vi "Main.vi"(8 "error in (no error)":errorcluster, 11 "ModuleAdmin":refnum<class "ModuleAdmin.lvclass">) -> ()   [LabVIEW 2014, in "AppModule.lvlib"]
uses:
  AppModule.lvlib
  <userlib>/NIST/ModuleAdminLib/ModuleAdmin/ModuleAdmin.lvclass
  PublicAPI/Arguments/Requests/clStopArgument.ctl
  <userlib>/NIST/BaseClasses/BasePlugin_class/BasePlugin.lvclass/BasePlugin.ctl
  AppPlugins/AppPluginBaseClass/AppPluginsBase.lvclass
  <userlib>/NIST/ModuleAdminLib/ModuleAdmin/ModuleAdmin.lvclass/ModuleAdmin.ctl
  Framework/FrontPanel/TypeDefs/clEventConfig.ctl
  Modules/EventPlugins/EventPluginBaseClass/TypeDefs/clEvtReportArray.ctl
  Modules/EventPlugins/EventPluginBaseClass/TypeDefs/clEvtReport.ctl
  AppPlugins/AppPluginBaseClass/AppPluginsBase.lvclass/AppPluginsBase.ctl
  PublicAPI/Arguments/Requests/BC_AppInfo.ctl
  Framework/BusController/Admin/Registry/BCReg.lvclass
  <vilib>/Utility/error.llb/DialogType.ctl
  <userlib>/NIST/BaseClasses/BasePlugin_class/Accessors/Read PluginIniFilePath.vi
  <userlib>/NIST/BaseClasses/BasePlugin_class/Accessors/Write PluginIniFilePath.vi
  <userlib>/NIST/ModuleAdminLib/ModuleAdmin/Accessors/Write ShowPanel_.vi
  AppPlugins/AppPluginBaseClass/Accessors/Write clEvtReportArray.vi
  AppPlugins/AppPluginBaseClass/Accessors/Read clEvtReportArray.vi
  AppPlugins/AppPluginBaseClass/Accessors/Write BC_AppInfo.vi
  AppPlugins/AppPluginBaseClass/Accessors/Read BC_AppInfo.vi
  <userlib>/NIST/ModuleAdminLib/ModuleAdmin/Accessors/Read ShowPanel_.vi
  <userlib>/NIST/ModuleAdminLib/ModuleAdmin/Accessors/Read CloneRegRef.vi
  <vilib>/Utility/error.llb/Error Cluster From Error Code.vi
  <vilib>/ErrorRing/Error Ring.xnode
  <userlib>/NIST/ModuleAdminLib/CloneRegistration/CloneRegistration.lvclass
  <userlib>/NIST/ModuleAdminLib/ModuleAdmin.lvlib
  <userlib>/NIST/BaseClasses/Object_class/BaseObject.lvclass
  Modules/EventPlugins/EventPluginBaseClass/EventPluginBaseClass.lvclass
  Framework/Framework.lvlib
panel:
  out "error out":errorcluster
  # "This is the template for your cloneable module.\nYou should modifiy this to perform the functionality\nthat you want it to perform"
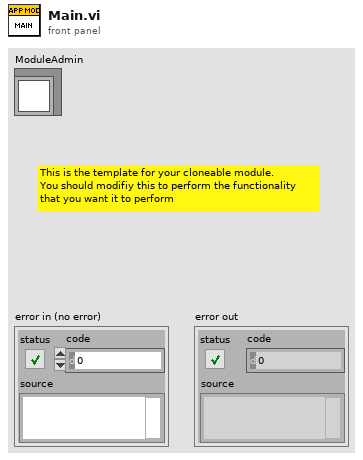
[diagram p1: front panel]
types:
  T1 = typedef "AppModule.lvlib/clRequestEvents.ctl" = cluster{"StopRequest":refnum<user-event>, "PathToINI":refnum<user-event>, " LoadPlugin":refnum<user-event>, "OpenAppConfig":refnum<user-event>, "WriteInputData":refnum<user-event>, "ReadInputData":refnum<user-event>, "GetAppOutput":refnum<user-event>, "WriteEvtConfig":refnum<user-event>, "WriteBcAppInfo":refnum<user-event>, "ReadBcAppInfo":refnum<user-event>, "AggregateRequest":refnum<user-event>, "WriteAppConfig":refnum<user-event>, "ReadAppConfig":refnum<user-event>, "CalcAppOutput":refnum<user-event>, "ShowPanel":refnum<user-event>}
  T2 = typedef "AppModule.lvlib/clBroadcastEvents.ctl" = cluster{"DidInit":refnum<user-event>, "StatusUpdate":refnum<user-event>, "ErrorReport":refnum<user-event>, "DidStop":refnum<user-event>, "PathToINI":refnum<user-event>, "InputData":refnum<user-event>, "OutputData":refnum<user-event>, "BcAppInfo":refnum<user-event>, "ConfigData":refnum<user-event>}
  T3 = typedef "AppModule.lvlib/clStopArgument.ctl" = cluster{"Exit via Stop Module Req?":bool, "Wait for Module to stop?":bool, "ModuleAdmin":refnum<class "ModuleAdmin.lvclass">}
  T4 = enum32{"Invalid", "Standard", "Closed", "Hidden", "Minimized", "Maximized"}
  T5 = typedef "Framework.lvlib/clEventConfig.ctl" = cluster{"UTC Time 0":timestamp, "Nominal Frequency":u16, "Reporting Rate":u16, "Fsamp":u32, "PosSeq":bool}
  T6 = typedef "EventPlugins.lvlib/EventPluginBaseClass.lvclass/clEvtReportArray.ctl" = T7[]
  T7 = typedef "EventPlugins.lvlib/EventPluginBaseClass.lvclass/clEvtReport.ctl" = cluster{"Timestamp":dbl, "Synx":cdb[], "Freq":dbl, "ROCOF":dbl, "ID":i16}
  T8 = typedef "AppModule.lvlib/BC_AppInfo.ctl" = cluster{"QueName":string, "BCRegRef":refnum<data-value>}
  T9 = typedef "DialogType.ctl" = u16
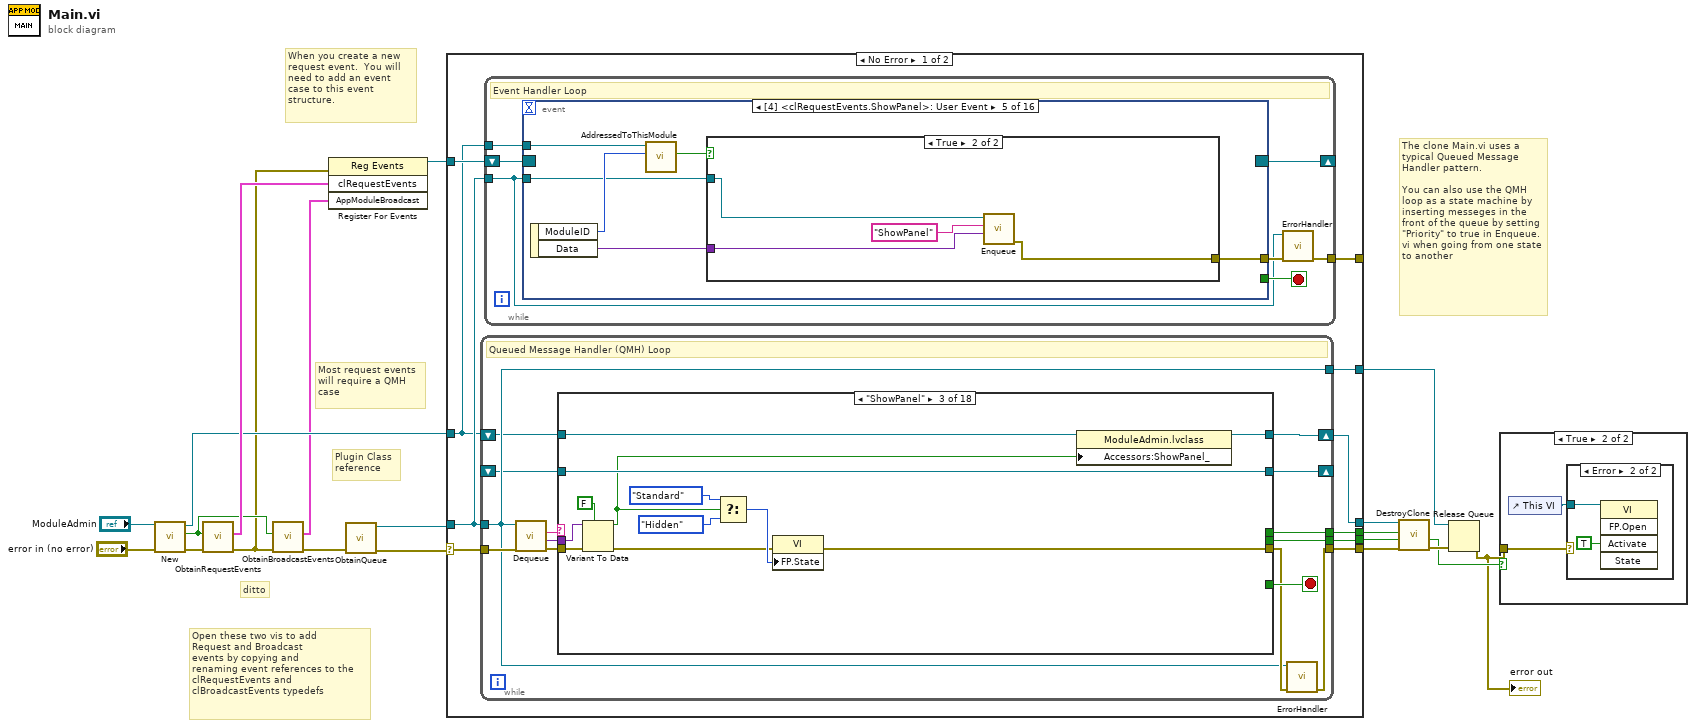
[diagram p0: block diagram]
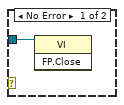
[diagram p3: hidden frame]
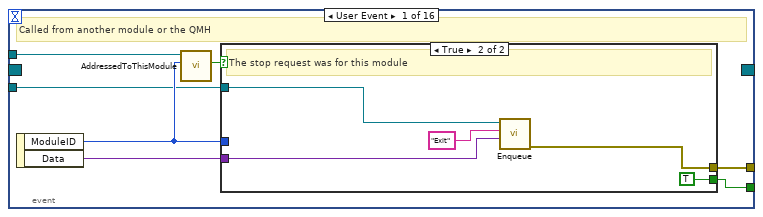
[diagram p4: hidden frame]
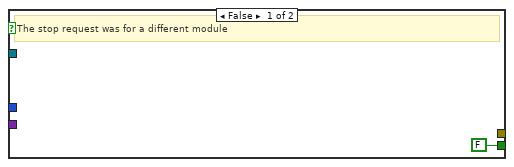
[diagram p5: hidden frame]
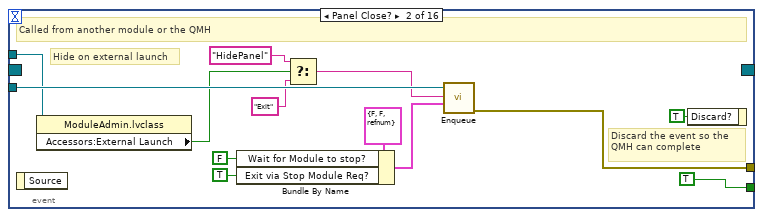
[diagram p6: hidden frame]
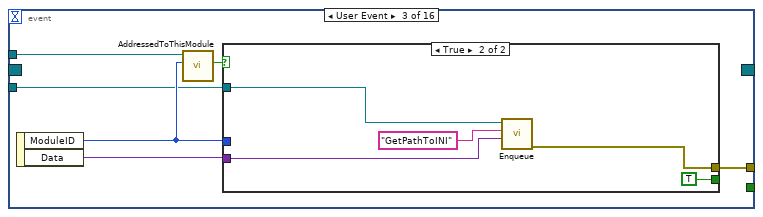
[diagram p7: hidden frame]
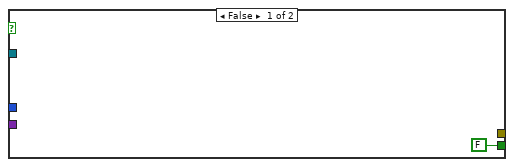
[diagram p8: hidden frame]
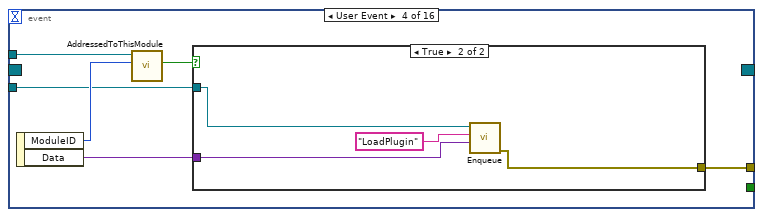
[diagram p9: hidden frame]
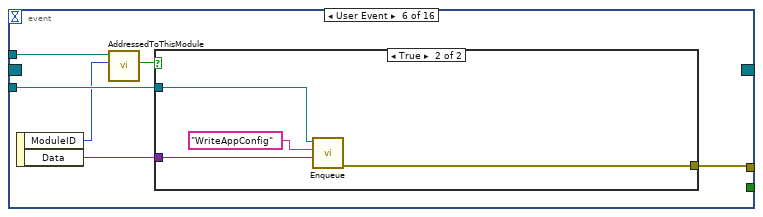
[diagram p12: hidden frame]
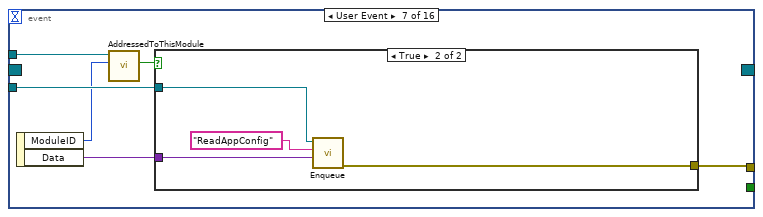
[diagram p14: hidden frame]
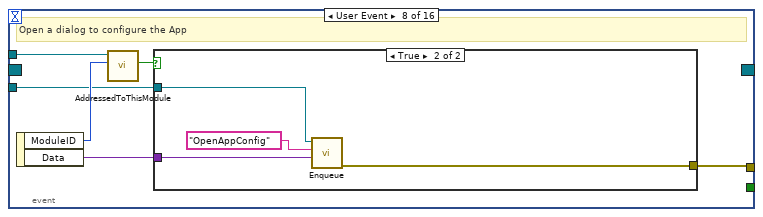
[diagram p16: hidden frame]
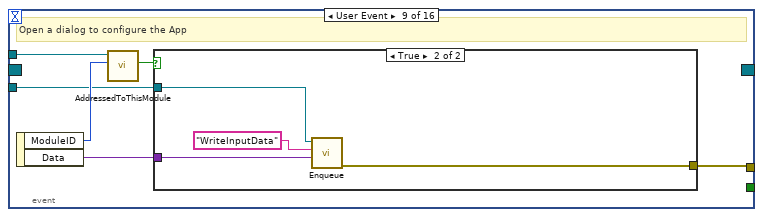
[diagram p18: hidden frame]
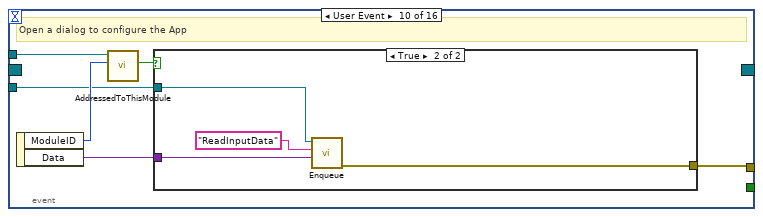
[diagram p20: hidden frame]
diagram:
  # "Plugin Class\nreference"
  # "The clone Main.vi uses a typical Queued Message Handler pattern.  \n\nYou can also use the QMH loop as a state machine by inserting messeges in the front of the queue by setting \"Priority\" to true in Enqueue.vi when going from one state to another"
  # "Open these two vis to add\nRequest and Broadcast \nevents by copying and \nrenaming event references to the \nclRequestEvents and \nclBroadcastEvents typedefs"
  # "ditto"
  # "Most request events\nwill require a QMH\ncase"
  # "When you create a new request event.  You will need to add an event case to this event structure."
  n1 = call <userlib>:"New.vi"("error in (no error)"="error in (no error)", "ModuleAdmin"="ModuleAdmin") -> ("error out"=w18:errorcluster, "First?"=w11:bool, "ModuleAdmin"=w14:refnum<class "ModuleAdmin.lvclass">)  [unwired: 7 in]
  n2 = call "ObtainRequestEvents.vi"("error in (no error)"=w18, "CreateNew (F)"=w11) -> ("error out"=w10:errorcluster, "clRequestEvents"=w17:T1)  [unwired: 8 in]
  n3 = call "ObtainBroadcastEvents.vi"("error in (no error)"=w10, "CreateNew? (F)"=w11) -> ("error out"=w12:errorcluster, "AppModuleBroadcast"=w9:T2)  [unwired: 8 in]
  n4 = register-events(error in=w10, w17, w9) -> (reference out=w8:refnum<event-registration>)  [unwired: 1 in, 1 out]
  n5 = call "ObtainQueue.vi"("error in (no error)"=w12) -> ("error out"=w16:errorcluster, "MessageQueue"=w15:refnum<queue>)  [unwired: 9 in]
  n6 = case shown="No Error" w16 {
    selector: w16 -> [w30 w473]
    tunnel: w15 -> [w28 w469]
    tunnel: w14 -> [w25 w470]
    tunnel: [w29 w471] -> w7
    tunnel: [w27 w469] -> w13
    tunnel: w8 -> [w26 _]
    tunnel: [w24 w468] -> w5
    tunnel: [w23 _] -> w4
    tunnel: [w22 _] -> w3
    tunnel: [w21 _] -> _
    frame No Error {
      n7 = while {
        tunnel: w28 -> [w210]
        tunnel: w30 -> [w218]
        tunnel: [w212] -> w29
        tunnel: [w210] -> w27
        tunnel: [w214] -> w23
        tunnel: [w213] -> w22
        shift-right: [w209] -> _
        shift-left: _ -> [w208]
        shift-right: [w206] -> w24
        shift-left: w25 -> [w207]
        stop <- w219 stop-if-true
        # "Queued Message Handler (QMH) Loop"
        n8 = call "Dequeue.vi"("error in (no error)"=w218, "MessageQueue"=w210) -> ("error out"=w217:errorcluster, "Message Data"=w215:variant, "Message"=w216:string)  [unwired: 6 in, 1 out]
        n9 = case shown="\"ShowPanel\"" w216 {
          selector: w216 -> [_ _ _ _ _ _ _ _ _ _ _ _ _ _ _ _ _ w454]
          tunnel: [_ _ _ _ _ _ _ _ _ _ _ _ _ _ _ TRUE _ _] -> w219
          tunnel: w207 -> [w226 w233 w276 w285 w299 w310 w311 w325 w340 w348 w363 w371 w384 w393 w414 w423 w434 w457]
          tunnel: [w227 w234 w278 w286 w296 w308 w315 w326 w336 w349 w360 w369 w380 w390 w403 w430 w435 w453] -> w211
          tunnel: w217 -> [w222 w243 w279 w289 w291 w305 w318 w331 w341 w354 w364 w373 w376 w388 _ w429 w443 _]
          tunnel: w215 -> [_ w245 w273 _ w292 _ w319 w330 _ w353 _ _ _ _ _ w428 w442 _]
          tunnel: [_ _ _ _ _ _ _ _ _ _ _ _ _ _ _ w426 _ _] -> w214
          tunnel: [_ _ _ _ _ _ _ _ _ _ _ _ _ _ _ w425 _ _] -> w213
          tunnel: [w223 w231 w277 w287 w295 w306 w314 w329 w339 w352 w362 w372 w378 w386 refnum<class "AppPluginsBase.lvclass"> refnum ("MyPlugins.lvlib:MyPluginsBase.lvclass") w424 w433 w451] -> w209
          tunnel: w208 -> [w225 w232 w277 w288 w294 w307 w317 w332 w342 w355 w365 w374 w377 w389 _ w424 w433 w451]
          tunnel: [w220 w229 w274 w285 w290 w300 w311 w320 w333 w343 w356 w366 w375 w385 w394 w423 w432 w450] -> w206
          frame "GetPathToINI" {
            n10 = property class="AppPluginsBase.lvclass"(reference=w225, error in=w222) -> (reference out=w223:refnum<class "AppPluginsBase.lvclass">, error out=w221:errorcluster, "Accessors:PluginIniFilePath"=w224:path)
            n11 = property class="ModuleAdmin.lvclass"(reference=w226) -> (reference out=w220:refnum<class "ModuleAdmin.lvclass">, "Accessors:Module ID"=w228:i32)  [unwired: 1 in, 1 out]
            n12 = call "PathToINIBroadcast.vi"("error in (no error)"=w221, "PathToINI"=w224, "ModuleID"=w228) -> ("error out"=w227:errorcluster)  [unwired: 8 in]
          }
          frame "LoadPlugin" {
            n13 = Variant To Data(error in=w243, type=path "", Variant=w245) -> (data=w230:path, error out=w242:errorcluster)
            n14 = call <userlib>:"GetPathToClass.vi"("error in (no error)"=w242, "configuration file path"=w230) -> ("error IO"=w238:errorcluster, "PathToClass"=w241:path)  [unwired: 8 in]
            n15 = Current VI's Path() -> (path=w240:path)
            n16 = Build Path(base path=w240, name or relative path=w241) -> (appended path=w239:path)
            n17 = call <vilib>:"Check if File or Folder Exists.vi"("error in (no error)"=w238, "path"=w239) -> ("error out"=w235:errorcluster, "file or folder exists?"=w237:bool, "dup path"=w236:path)  [unwired: 7 in]
            n18 = case shown="True" w237 {
              tunnel: w236 -> [w249 w263]
              tunnel: w235 -> [_ w272]
              tunnel: [w248 w267] -> w234
              tunnel: w233 -> [w246 w266]
              tunnel: w232 -> [w247 _]
              tunnel: [w247 w260] -> w231
              tunnel: w230 -> [_ w259]
              tunnel: [w246 w258] -> w229
              frame False {
                n19 = Path To String(path=w249) -> (string=w250:string)
                n20 = xnode "Error Ring"("parameter 0"=w250) -> ("error out"=w248:errorcluster)
              }
              frame True {
                n21 = call-dynamic "LoadClassFromFile.vi"("error in (no error)"=w272, "class path"=w263, "reference in"=refnum<class "AppPluginsBase.lvclass"> refnum ("MyPlugins.lvlib:MyPluginsBase.lvclass")) -> ("error out"=w262:errorcluster, "reference out"=w264:refnum<class "AppPluginsBase.lvclass">)  [unwired: 7 in]
                n22 = property class="ModuleAdmin.lvclass"(reference=w266) -> (reference out=w258:refnum<class "ModuleAdmin.lvclass">, "Accessors:Module ID"=w265:i32)  [unwired: 1 in, 1 out]
                n23 = property class="AppPluginsBase.lvclass"(reference=w264, error in=w262, "Accessors:PluginIniFilePath"=w259) -> (reference out=w260:refnum<class "AppPluginsBase.lvclass">, error out=w261:errorcluster)
                n24 = Path To String(path=w263) -> (string=w269:string)
                n25 = Format Into String(format string="Plugin %s loaded ", w269) -> (resulting string=w268:string)  [unwired: 2 in, 1 out]
                n26 = call "StatusUpdate.vi"("error in (no error)"=w261, "Status"=w268, "ModuleID"=w265) -> ("error out"=w267:errorcluster)  [unwired: 8 in]
              }
            }
          }
          frame "ShowPanel" {
            n27 = Variant To Data(error in=w279, type=FALSE, Variant=w273) -> (data=w275:bool, error out=w281:errorcluster)
            n28 = Select(t=T4."Standard" ("Front Panel Window:State"), s=w275, f=T4."Hidden" ("Front Panel Window:State")) -> (s? t:f=w284:T4)
            n29 = property class="VI"(error in=w281, "FP.State"=w284) -> (error out=w278:errorcluster)  [unwired: 1 in, 1 out]
            n30 = property class="ModuleAdmin.lvclass"(reference=w276, "Accessors:ShowPanel_"=w275) -> (reference out=w274:refnum<class "ModuleAdmin.lvclass">)  [unwired: 1 in, 1 out]
          }
          frame "OpenAppConfig" {
            n31 = call-dynamic "AppConfig.vi"("error in (no error)"=w289, "AppPluginsBase"=w288) -> ("error out"=w286:errorcluster, "AppPluginsBase out"=w287:refnum<class "AppPluginsBase.lvclass">)  [unwired: 8 in]
          }
          frame "WriteAppConfig" {
            n32 = call-dynamic "AppConfigXMLToType.vi"("error in (no error)"=w291, "Config in"=w292, "AppPluginsBase in"=w294) -> ("error out"=w293:errorcluster, "AppPluginsBase out"=w295:refnum<class "AppPluginsBase.lvclass">)  [unwired: 7 in]
            n33 = property class="ModuleAdmin.lvclass"(reference=w299) -> (reference out=w290:refnum<class "ModuleAdmin.lvclass">, "Accessors:Module ID"=w298:i32)  [unwired: 1 in, 1 out]
            n34 = call "StatusUpdate.vi"("error in (no error)"=w293, "Status"="App Config Received", "ModuleID"=w298) -> ("error out"=w296:errorcluster)  [unwired: 8 in]
          }
          frame "ReadAppConfig" {
            n35 = property class="ModuleAdmin.lvclass"(reference=w310) -> (reference out=w300:refnum<class "ModuleAdmin.lvclass">, "Accessors:Module ID"=w301:i32)  [unwired: 1 in, 1 out]
            n36 = call-dynamic "AppConfigTypeToXML.vi"("error in (no error)"=w305, "AppPluginsBase in"=w307) -> ("error out"=w304:errorcluster, "ConfigXML out"=w302:string, "AppPluginsBase out"=w306:refnum<class "AppPluginsBase.lvclass">)  [unwired: 7 in]
            n37 = call "ConfigData.vi"("error in (no error)"=w304, "CfgXML in"=w302, "ModuleID"=w301) -> ("error out"=w303:errorcluster)  [unwired: 8 in]
            n38 = call "StatusUpdate.vi"("error in (no error)"=w303, "Status"="App Config Transmitted", "ModuleID"=w301) -> ("error out"=w308:errorcluster)  [unwired: 8 in]
          }
          frame "WriteEvtConfig" {
            n39 = Variant To Data(error in=w318, type=T5 {"UTC Time 0"=timestamp(0 s since 1904-01-01), "Nominal Frequency"=60, "Reporting Rate"=60, "Fsamp"=960, "PosSeq"=FALSE} ("Event Configuration"), Variant=w319) -> (data=w312:T5, error out=w316:errorcluster)
            n40 = call-dynamic "WriteEvtConfig.vi"("error in (no error)"=w316, "Event Configuration"=w312, "AppPluginsBase in"=w317) -> ("error out"=w315:errorcluster, "AppPluginsBase out"=w314:refnum<class "AppPluginsBase.lvclass">)  [unwired: 7 in]
          }
          frame "WriteInputData" {
            n41 = Variant To Data(error in=w331, type=T6 [] ("clEvtReportArray"), Variant=w330) -> (data=w321:T6, error out=w328:errorcluster)
            n42 = property class="AppPluginsBase.lvclass"(reference=w332, error in=w328, "Accessors:clEvtReportArray"=w321) -> (reference out=w329:refnum<class "AppPluginsBase.lvclass">, error out=w327:errorcluster)
            n43 = property class="ModuleAdmin.lvclass"(reference=w325) -> (reference out=w320:refnum<class "ModuleAdmin.lvclass">, "Accessors:Module ID"=w324:i32)  [unwired: 1 in, 1 out]
            n44 = call "StatusUpdate.vi"("error in (no error)"=w327, "Status"="Received App Input Data", "ModuleID"=w324) -> ("error out"=w326:errorcluster)  [unwired: 8 in]
          }
          frame "ReadInputData" {
            n45 = property class="AppPluginsBase.lvclass"(reference=w342) -> (reference out=w339:refnum<class "AppPluginsBase.lvclass">, "Accessors:clEvtReportArray"=w338:T6)  [unwired: 1 in, 1 out]
            n46 = property class="ModuleAdmin.lvclass"(reference=w340) -> (reference out=w333:refnum<class "ModuleAdmin.lvclass">, "Accessors:Module ID"=w335:i32)  [unwired: 1 in, 1 out]
            n47 = call "InputData.vi"("error in (no error)"=w341, "clEvtReportArray in"=w338, "ModuleID"=w335) -> ("error out"=w337:errorcluster)  [unwired: 8 in]
            n48 = call "StatusUpdate.vi"("error in (no error)"=w337, "Status"="Transmitted Input Data", "ModuleID"=w335) -> ("error out"=w336:errorcluster)  [unwired: 8 in]
          }
          frame "WriteBcAppInfo" {
            n49 = Variant To Data(error in=w354, type=T8 {"QueName"="", "BCRegRef"=refnum} ("BC_AppInfo"), Variant=w353) -> (data=w345:T8, error out=w351:errorcluster)
            n50 = property class="AppPluginsBase.lvclass"(reference=w355, error in=w351, "Accessors:BC_AppInfo"=w345) -> (reference out=w352:refnum<class "AppPluginsBase.lvclass">, error out=w350:errorcluster)
            n51 = property class="ModuleAdmin.lvclass"(reference=w348) -> (reference out=w343:refnum<class "ModuleAdmin.lvclass">, "Accessors:Module ID"=w347:i32)  [unwired: 1 in, 1 out]
            n52 = call "StatusUpdate.vi"("error in (no error)"=w350, "Status"="Received Bus Controller Info", "ModuleID"=w347) -> ("error out"=w349:errorcluster)  [unwired: 8 in]
          }
          frame "ReadBcAppInfo" {
            n53 = property class="AppPluginsBase.lvclass"(reference=w365) -> (reference out=w362:refnum<class "AppPluginsBase.lvclass">, "Accessors:BC_AppInfo"=w357:T8)  [unwired: 1 in, 1 out]
            n54 = property class="ModuleAdmin.lvclass"(reference=w363) -> (reference out=w356:refnum<class "ModuleAdmin.lvclass">, "Accessors:Module ID"=w359:i32)  [unwired: 1 in, 1 out]
            n55 = call "BcAppInfo.vi"("error in (no error)"=w364, "AppOutputData"=w357, "ModuleID"=w359) -> ("error out"=w361:errorcluster)  [unwired: 8 in]
            n56 = call "StatusUpdate.vi"("error in (no error)"=w361, "Status"="Transmitted Bus Controller Info", "ModuleID"=w359) -> ("error out"=w360:errorcluster)  [unwired: 8 in]
          }
          frame "Aggregate" {
            n57 = call-dynamic "Aggregate.vi"("ModuleAdmin"=w371, "error in (no error)"=w373, "AppPluginsBase in"=w374) -> ("error out"=w370:errorcluster, "AppPluginsBase out"=w372:refnum<class "AppPluginsBase.lvclass">)  [unwired: 7 in]
            n58 = property class="ModuleAdmin.lvclass"(reference=w371) -> (reference out=w366:refnum<class "ModuleAdmin.lvclass">, "Accessors:Module ID"=w368:i32)  [unwired: 1 in, 1 out]
            n59 = call "StatusUpdate.vi"("error in (no error)"=w370, "Status"="Appmodule Aggregate Complete", "ModuleID"=w368) -> ("error out"=w369:errorcluster)  [unwired: 8 in]
          }
          frame "GetOutputData" {
            n60 = property class="ModuleAdmin.lvclass"(reference=w384) -> (reference out=w375:refnum<class "ModuleAdmin.lvclass">, "Accessors:Module ID"=w383:i32)  [unwired: 1 in, 1 out]
            n61 = property class="AppPluginsBase.lvclass"(reference=w377) -> (reference out=w378:refnum<class "AppPluginsBase.lvclass">, "Accessors:AppOutputData"=w379:variant)  [unwired: 1 in, 1 out]
            n62 = call "OutputData.vi"("error in (no error)"=w376, "AppOutputData"=w379, "ModuleID"=w383) -> ("error out"=w382:errorcluster)  [unwired: 8 in]
            n63 = call "StatusUpdate.vi"("error in (no error)"=w382, "Status"="Transmitted Output Data", "ModuleID"=w383) -> ("error out"=w380:errorcluster)  [unwired: 8 in]
          }
          frame "CalcAppOutput" {
            n64 = property class="ModuleAdmin.lvclass"(reference=w393) -> (reference out=w385:refnum<class "ModuleAdmin.lvclass">, "Accessors:Module ID"=w392:i32)  [unwired: 1 in, 1 out]
            n65 = call-dynamic "GetAppOutput.vi"("error in (no error)"=w388, "AppPluginsBase in"=w389) -> ("error out"=w387:errorcluster, "AppPluginsBase out"=w386:refnum<class "AppPluginsBase.lvclass">)  [unwired: 8 in]
            n66 = call "StatusUpdate.vi"("error in (no error)"=w387, "Status"="Calculated Output Data", "ModuleID"=w392) -> ("error out"=w390:errorcluster)  [unwired: 8 in]
          }
          frame "Initialize" {
            # "Initialize is always called after ObtainQueue.vi is run"
            n67 = property class="ModuleAdmin.lvclass"(reference=w414) -> (reference out=w400:refnum<class "ModuleAdmin.lvclass">, error out=w411:errorcluster, "Accessors:Module ID"=w402:i32, "Accessors:ShowPanel_"=w397:bool, "Accessors:External Launch"=w396:bool, "Accessors:ModuleName"=w398:string)  [unwired: 1 in]
            n68 = Compound Arithmetic op=OR(w397, invert w396) -> (w395:bool)
            n69 = Select(t=T4."Standard" ("Front Panel Window:State"), s=w395, f=T4."Hidden" ("Front Panel Window:State")) -> (s? t:f=w407:T4)
            n70 = invoke class="VI" method="FP.Open"(error in=w411, "State"=w407) -> (error out=w410:errorcluster)  [unwired: 3 in, 4 out]
            n71 = call <userlib>:"ModuleName.vi"("Name"=w398, "ModuleID"=w402) -> ("ModuleName"=w406:string)  [unwired: 9 in]
            n72 = property class="VI"(error in=w410, "Front Panel.Title"=w406) -> (reference out=w413:refnum<vi>, error out=w412:errorcluster)  [unwired: 1 in]
            n73 = invoke class="VI" method="FP.Center"(reference=w413, error in=w412) -> (error out=w401:errorcluster)  [unwired: 1 in, 2 out]
            n74 = case shown="True" w396 {
              tunnel: [w415 w421] -> w404
              tunnel: [w416 w418] -> w394
              tunnel: w401 -> [w415 w420]
              tunnel: w400 -> [w416 w417]
              frame False {
              }
              frame True {
                n75 = call <userlib>:"WaitOnModuleSync.vi"("error in (no error)"=w420, "ModuleAdmin"=w417) -> ("error out"=w422:errorcluster, "ModuleAdmin"=w419:refnum<class "ModuleAdmin.lvclass">)  [unwired: 8 in]
                n76 = call <userlib>:"WaitOnEventSync.vi"("error in (no error)"=w422, "ModuleAdmin"=w419) -> ("error out"=w421:errorcluster, "ModuleAdmin"=w418:refnum<class "ModuleAdmin.lvclass">)  [unwired: 8 in]
              }
            }
            n77 = call "DidInit.vi"("Init?"=TRUE, "error in (no error)"=w404, "ModuleAdmin"=w394) -> ("error out"=w403:errorcluster)  [unwired: 8 in]
          }
          frame "Exit" {
            # "Called by the StopRequest event handler case"
            n78 = control-ref of="This VI"() -> (w427:refnum<vi>)
            n79 = call "HandleExit.vi"("error in (no error)"=w429, "VI Refnum"=w427, "StopArgument"=w428, "ModuleAdmin"=w423) -> ("error out"=w430:errorcluster, "Exit via Stop Module Req?"=w425:bool, "WaitForStop?"=w426:bool)  [unwired: 5 in]
          }
          frame "Error" {
            n80 = property class="ModuleAdmin.lvclass"(reference=w434) -> ("Accessors:External Launch"=w438:bool, "Accessors:Module ID"=w436:i32)  [unwired: 1 in, 2 out]
            n81 = Variant To Data(error in=w443, type=errorcluster {"status"=FALSE, "code"=0, "source"=""} ("error constant"), Variant=w442) -> (data=w437:errorcluster, error out=w440:errorcluster)
            n82 = call "ReportError.vi"("error in (no error)"=w440, "ErrorReported"=w437, "ModuleID"=w436) -> ("error out"=w439:errorcluster)  [unwired: 8 in]
            n83 = case shown="True" w438 {
              tunnel: w439 -> [w447 w449]
              tunnel: w437 -> [w446 _]
              tunnel: [w445 w449] -> w435
              tunnel: w434 -> [w444 w448]
              tunnel: [w444 w448] -> w432
              frame False {
                # "Todo:  Add an event to ask the user\nIf the module should stop or continue"
                # "Stand alone: now, force an exit"
                n84 = call <vilib>:"Simple Error Handler.vi"("error in (no error)"=w446) -> ()  [unwired: 4 in, 5 out]
                n85 = call "StopRequest.vi"("error in (no error)"=w447, "ModuleAdmin"=w444) -> ("error out"=w445:errorcluster)  [unwired: 8 in, 1 out]
              }
              frame True {
                # "Externally launched modules only broadcast the error msg"
              }
            }
          }
          frame Default {
            # "Called only if a message was queued and no QMH case was created"
            n86 = property class="ModuleAdmin.lvclass"(reference=w457) -> (reference out=w450:refnum<class "ModuleAdmin.lvclass">, "Accessors:Module ID"=w456:i32, "Accessors:ModuleName"=w452:string)  [unwired: 1 in, 1 out]
            n87 = call <userlib>:"ModuleName.vi"("Name"=w452, "ModuleID"=w456) -> ("ModuleName"=w455:string)  [unwired: 9 in]
            n88 = xnode "Error Ring"("parameter 0"=w454, "parameter 1"=w455) -> ("error out"=w453:errorcluster)
          }
        }
        n89 = call "ErrorHandler.vi"("error in (no error)"=w211, "MessageQueue"=w210) -> ("error out"=w212:errorcluster)  [unwired: 8 in, 1 out]
      }
      n90 = while {
        tunnel: w28 -> [w31]
        shift-right: [w35] -> _
        shift-left: w26 -> [w36]
        tunnel: w25 -> [w34]
        tunnel: [w32] -> w21
        stop <- w37 stop-if-true
        # "Event Handler Loop"
        n91 = event shown="[4] <clRequestEvents.ShowPanel>: User Event" {
          selector: w36 -> [_ _ _ _ _ _ _ _ _ _ _ _ _ _ _ _]
          dyn-events: [_ _ _ _ _ _ _ _ _ _ _ _ _ _ _ _] -> w35
          timeout: _ -> [_ _ _ _ _ _ _ _ _ _ _ _ _ _ _ _]
          tunnel: w31 -> [w41 w63 w66 w77 w87 w99 w109 w119 w129 w139 w149 w159 w169 w179 w189 w199]
          tunnel: [w40 TRUE _ _ _ _ _ _ _ _ _ _ _ _ _ _] -> w37
          tunnel: w34 -> [w44 w57 w65 w81 w91 w100 w110 w120 w130 w140 w150 w160 w170 w180 w190 w200]
          tunnel: [w39 w61 w64 w78 w88 w96 w106 w116 w126 w136 w146 w156 w166 w176 w186 w196] -> w33
          event User Event {
            # "Called from another module or the QMH"
            n92 = event-data() -> ("ModuleID"=w42:i32, "Data"=w38:variant)  [unwired: 1 in]
            n93 = call <userlib>:"AddressedToThisModule.vi"("ModuleID"=w42, "ModuleAdmin"=w44) -> ("AddressedToThisInstance?"=w43:bool)  [unwired: 8 in, 1 out]
            n94 = case shown="True" w43 {
              tunnel: w42 -> [_ _]
              tunnel: w41 -> [_ w50]
              tunnel: [FALSE TRUE] -> w40
              tunnel: [_ w48] -> w39
              tunnel: w38 -> [_ w46]
              frame False {
                # "The stop request was for a different module"
              }
              frame True {
                # "The stop request was for this module"
                n95 = call "Enqueue.vi"("Message Data"=w46, "Message"="Exit", "MessageQueue"=w50) -> ("error out"=w48:errorcluster)  [unwired: 7 in, 1 out]
              }
            }
          }
          event Panel Close? {
            # "Hide on external launch"
            # "Discard the event so the QMH can complete"
            # "Called from another module or the QMH"
            n96 = event-data() -> ()  [unwired: 1 in, 1 out]
            n97 = property class="ModuleAdmin.lvclass"(reference=w57) -> ("Accessors:External Launch"=w52:bool)  [unwired: 1 in, 2 out]
            n98 = Bundle By Name(cluster=T3 {"Exit via Stop Module Req?"=FALSE, "Wait for Module to stop?"=FALSE, "ModuleAdmin"=refnum} ("Stop Argument"), "Wait for Module to stop?"=FALSE, "Exit via Stop Module Req?"=TRUE) -> (w58:T3)
            n99 = Select(t="HidePanel", s=w52, f="Exit" ("Message")) -> (s? t:f=w54:string)
            n100 = call "Enqueue.vi"("Message Data"=w58, "Message"=w54, "MessageQueue"=w63) -> ("error out"=w61:errorcluster)  [unwired: 7 in, 1 out]
            n101 = event-data("Discard?"=TRUE) -> ()  [unwired: 1 in, 1 out]
          }
          event User Event {
            n102 = event-data() -> ("ModuleID"=w67:i32, "Data"=w68:variant)  [unwired: 1 in]
            n103 = call <userlib>:"AddressedToThisModule.vi"("ModuleID"=w67, "ModuleAdmin"=w65) -> ("AddressedToThisInstance?"=w69:bool)  [unwired: 8 in, 1 out]
            n104 = case shown="True" w69 {
              tunnel: w67 -> [_ _]
              tunnel: w66 -> [_ w75]
              tunnel: [FALSE TRUE] -> _
              tunnel: [_ w73] -> w64
              tunnel: w68 -> [_ w71]
              frame False {
                # "The stop request was for a different module"
              }
              frame True {
                # "The stop request was for this module"
                n105 = call "Enqueue.vi"("Message Data"=w71, "Message"="GetPathToINI", "MessageQueue"=w75) -> ("error out"=w73:errorcluster)  [unwired: 7 in, 1 out]
              }
            }
          }
          event User Event {
            n106 = event-data() -> ("ModuleID"=w80:i32, "Data"=w76:variant)  [unwired: 1 in]
            n107 = call <userlib>:"AddressedToThisModule.vi"("ModuleID"=w80, "ModuleAdmin"=w81) -> ("AddressedToThisInstance?"=w79:bool)  [unwired: 8 in, 1 out]
            n108 = case shown="True" w79 {
              tunnel: [_ w82] -> w78
              tunnel: w77 -> [_ w85]
              tunnel: w76 -> [_ w83]
              frame False {
              }
              frame True {
                n109 = call "Enqueue.vi"("Message Data"=w83, "Message"="LoadPlugin", "MessageQueue"=w85) -> ("error out"=w82:errorcluster)  [unwired: 7 in, 1 out]
              }
            }
          }
          event User Event {
            n110 = event-data() -> ("ModuleID"=w90:i32, "Data"=w86:variant)  [unwired: 1 in]
            n111 = call <userlib>:"AddressedToThisModule.vi"("ModuleID"=w90, "ModuleAdmin"=w91) -> ("AddressedToThisInstance?"=w89:bool)  [unwired: 8 in, 1 out]
            n112 = case shown="True" w89 {
              tunnel: [_ w92] -> w88
              tunnel: w87 -> [_ w95]
              tunnel: w86 -> [_ w93]
              frame False {
              }
              frame True {
                n113 = call "Enqueue.vi"("Message Data"=w93, "Message"="ShowPanel", "MessageQueue"=w95) -> ("error out"=w92:errorcluster)  [unwired: 7 in, 1 out]
              }
            }
          }
          event User Event {
            n114 = event-data() -> ("ModuleID"=w98:i32, "Data"=w97:variant)  [unwired: 1 in]
            n115 = call <userlib>:"AddressedToThisModule.vi"("ModuleID"=w98, "ModuleAdmin"=w100) -> ("AddressedToThisInstance?"=w101:bool)  [unwired: 8 in, 1 out]
            n116 = case shown="True" w101 {
              tunnel: w99 -> [_ w103]
              tunnel: w97 -> [_ w105]
              tunnel: [_ w102] -> w96
              frame False {
              }
              frame True {
                n117 = call "Enqueue.vi"("Message Data"=w105, "Message"="WriteAppConfig", "MessageQueue"=w103) -> ("error out"=w102:errorcluster)  [unwired: 7 in, 1 out]
              }
            }
          }
          event User Event {
            n118 = event-data() -> ("ModuleID"=w108:i32, "Data"=w107:variant)  [unwired: 1 in]
            n119 = call <userlib>:"AddressedToThisModule.vi"("ModuleID"=w108, "ModuleAdmin"=w110) -> ("AddressedToThisInstance?"=w111:bool)  [unwired: 8 in, 1 out]
            n120 = case shown="True" w111 {
              tunnel: w109 -> [_ w113]
              tunnel: w107 -> [_ w115]
              tunnel: [_ w112] -> w106
              frame False {
              }
              frame True {
                n121 = call "Enqueue.vi"("Message Data"=w115, "Message"="ReadAppConfig", "MessageQueue"=w113) -> ("error out"=w112:errorcluster)  [unwired: 7 in, 1 out]
              }
            }
          }
          event User Event {
            # "Open a dialog to configure the App"
            n122 = event-data() -> ("ModuleID"=w121:i32, "Data"=w117:variant)  [unwired: 1 in]
            n123 = call <userlib>:"AddressedToThisModule.vi"("ModuleID"=w121, "ModuleAdmin"=w120) -> ("AddressedToThisInstance?"=w118:bool)  [unwired: 8 in, 1 out]
            n124 = case shown="True" w118 {
              tunnel: w119 -> [_ w123]
              tunnel: w117 -> [_ w125]
              tunnel: [_ w122] -> w116
              frame False {
              }
              frame True {
                n125 = call "Enqueue.vi"("Message Data"=w125, "Message"="OpenAppConfig", "MessageQueue"=w123) -> ("error out"=w122:errorcluster)  [unwired: 7 in, 1 out]
              }
            }
          }
          event User Event {
            # "Open a dialog to configure the App"
            n126 = event-data() -> ("ModuleID"=w131:i32, "Data"=w127:variant)  [unwired: 1 in]
            n127 = call <userlib>:"AddressedToThisModule.vi"("ModuleID"=w131, "ModuleAdmin"=w130) -> ("AddressedToThisInstance?"=w128:bool)  [unwired: 8 in, 1 out]
            n128 = case shown="True" w128 {
              tunnel: w129 -> [_ w133]
              tunnel: w127 -> [_ w135]
              tunnel: [_ w132] -> w126
              frame False {
              }
              frame True {
                n129 = call "Enqueue.vi"("Message Data"=w135, "Message"="WriteInputData", "MessageQueue"=w133) -> ("error out"=w132:errorcluster)  [unwired: 7 in, 1 out]
              }
            }
          }
          event User Event {
            # "Open a dialog to configure the App"
            n130 = event-data() -> ("ModuleID"=w141:i32, "Data"=w137:variant)  [unwired: 1 in]
            n131 = call <userlib>:"AddressedToThisModule.vi"("ModuleID"=w141, "ModuleAdmin"=w140) -> ("AddressedToThisInstance?"=w138:bool)  [unwired: 8 in, 1 out]
            n132 = case shown="True" w138 {
              tunnel: w139 -> [_ w143]
              tunnel: w137 -> [_ w145]
              tunnel: [_ w142] -> w136
              frame False {
              }
              frame True {
                n133 = call "Enqueue.vi"("Message Data"=w145, "Message"="ReadInputData", "MessageQueue"=w143) -> ("error out"=w142:errorcluster)  [unwired: 7 in, 1 out]
              }
            }
          }
          event User Event {
            # "Open a dialog to configure the App"
            n134 = event-data() -> ("ModuleID"=w151:i32, "Data"=w147:variant)  [unwired: 1 in]
            n135 = call <userlib>:"AddressedToThisModule.vi"("ModuleID"=w151, "ModuleAdmin"=w150) -> ("AddressedToThisInstance?"=w148:bool)  [unwired: 8 in, 1 out]
            n136 = case shown="True" w148 {
              tunnel: w149 -> [_ w153]
              tunnel: w147 -> [_ w155]
              tunnel: [_ w152] -> w146
              frame False {
              }
              frame True {
                n137 = call "Enqueue.vi"("Message Data"=w155, "Message"="GetOutputData", "MessageQueue"=w153) -> ("error out"=w152:errorcluster)  [unwired: 7 in, 1 out]
              }
            }
          }
          event User Event {
            # "Open a dialog to configure the App"
            n138 = event-data() -> ("ModuleID"=w161:i32, "Data"=w157:variant)  [unwired: 1 in]
            n139 = call <userlib>:"AddressedToThisModule.vi"("ModuleID"=w161, "ModuleAdmin"=w160) -> ("AddressedToThisInstance?"=w158:bool)  [unwired: 8 in, 1 out]
            n140 = case shown="True" w158 {
              tunnel: w159 -> [_ w163]
              tunnel: w157 -> [_ w165]
              tunnel: [_ w162] -> w156
              frame False {
              }
              frame True {
                n141 = call "Enqueue.vi"("Message Data"=w165, "Message"="CalcAppOutput", "MessageQueue"=w163) -> ("error out"=w162:errorcluster)  [unwired: 7 in, 1 out]
              }
            }
          }
          event User Event {
            # "Open a dialog to configure the App"
            n142 = event-data() -> ("ModuleID"=w171:i32, "Data"=w167:variant)  [unwired: 1 in]
            n143 = call <userlib>:"AddressedToThisModule.vi"("ModuleID"=w171, "ModuleAdmin"=w170) -> ("AddressedToThisInstance?"=w168:bool)  [unwired: 8 in, 1 out]
            n144 = case shown="True" w168 {
              tunnel: w169 -> [_ w173]
              tunnel: w167 -> [_ w175]
              tunnel: [_ w172] -> w166
              frame False {
              }
              frame True {
                n145 = call "Enqueue.vi"("Message Data"=w175, "Message"="WriteEvtConfig", "MessageQueue"=w173) -> ("error out"=w172:errorcluster)  [unwired: 7 in, 1 out]
              }
            }
          }
          event User Event {
            # "Open a dialog to configure the App"
            n146 = event-data() -> ("ModuleID"=w181:i32, "Data"=w177:variant)  [unwired: 1 in]
            n147 = call <userlib>:"AddressedToThisModule.vi"("ModuleID"=w181, "ModuleAdmin"=w180) -> ("AddressedToThisInstance?"=w178:bool)  [unwired: 8 in, 1 out]
            n148 = case shown="True" w178 {
              tunnel: w179 -> [_ w183]
              tunnel: w177 -> [_ w185]
              tunnel: [_ w182] -> w176
              frame False {
              }
              frame True {
                n149 = call "Enqueue.vi"("Message Data"=w185, "Message"="WriteBcAppInfo", "MessageQueue"=w183) -> ("error out"=w182:errorcluster)  [unwired: 7 in, 1 out]
              }
            }
          }
          event User Event {
            # "Open a dialog to configure the App"
            n150 = event-data() -> ("ModuleID"=w191:i32, "Data"=w187:variant)  [unwired: 1 in]
            n151 = call <userlib>:"AddressedToThisModule.vi"("ModuleID"=w191, "ModuleAdmin"=w190) -> ("AddressedToThisInstance?"=w188:bool)  [unwired: 8 in, 1 out]
            n152 = case shown="True" w188 {
              tunnel: w189 -> [_ w193]
              tunnel: w187 -> [_ w195]
              tunnel: [_ w192] -> w186
              frame False {
              }
              frame True {
                n153 = call "Enqueue.vi"("Message Data"=w195, "Message"="ReadBcAppInfo", "MessageQueue"=w193) -> ("error out"=w192:errorcluster)  [unwired: 7 in, 1 out]
              }
            }
          }
          event User Event {
            # "Open a dialog to configure the App"
            n154 = event-data() -> ("ModuleID"=w201:i32, "Data"=w197:variant)  [unwired: 1 in]
            n155 = call <userlib>:"AddressedToThisModule.vi"("ModuleID"=w201, "ModuleAdmin"=w200) -> ("AddressedToThisInstance?"=w198:bool)  [unwired: 8 in, 1 out]
            n156 = case shown="True" w198 {
              tunnel: w199 -> [_ w203]
              tunnel: w197 -> [_ w205]
              tunnel: [_ w202] -> w196
              frame False {
              }
              frame True {
                n157 = call "Enqueue.vi"("Message Data"=w205, "Message"="Aggregate", "MessageQueue"=w203) -> ("error out"=w202:errorcluster)  [unwired: 7 in, 1 out]
              }
            }
          }
        }
        n158 = call "ErrorHandler.vi"("error in (no error)"=w33, "MessageQueue"=w31) -> ("error out"=w32:errorcluster)  [unwired: 8 in, 1 out]
      }
    }
    frame Error {
      n159 = property class="ModuleAdmin.lvclass"(reference=w470) -> (reference out=w468:refnum<class "ModuleAdmin.lvclass">, "Accessors:CloneRegRef"=w467:refnum<data-value>, "Accessors:Module ID"=w466:i32)  [unwired: 1 in, 1 out]
      n160 = call <userlib>:"Remove.vi"("Module ID"=w466, "CloneRegRef"=w467) -> ("error out"=w472:errorcluster)  [unwired: 7 in, 2 out]
      n161 = flat-sequence {
        tunnel: w473 -> [w476]
        tunnel: w472 -> [_]
        tunnel: [w474] -> w471
        frame #0 {
          w475 = T9 2 items=["no dialog", "OK message", "continue or stop message", "OK message + warnings", "continue/stop + warnings"] ("type of dialog (OK msg:1)")
          n162 = call <vilib>:"Simple Error Handler.vi"("type of dialog (OK msg:1)"=w475, "error in (no error)"=w476) -> ("error out"=w474:errorcluster)  [unwired: 3 in, 4 out]
        }
      }
    }
  }
  n163 = call "DestroyClone.vi"("error in (no error)"=w7, "Exit via Stop Module Req?"=w3, "Wait for Module to stop?"=w4, "ModuleAdmin"=w5) -> ("error out"=w6:errorcluster, "External Launch"=w2:bool)  [unwired: 5 in, 1 out]
  n164 = Release Queue(queue=w13, error in (no error)=w6) -> (error out=w1:errorcluster)  [unwired: 1 in, 2 out]
  "error out" <- w1
  n165 = case shown="True" w2 {
    tunnel: w1 -> [_ w478]
    frame False {
    }
    frame True {
      n166 = control-ref of="This VI"() -> (w477:refnum<vi>)
      n167 = case shown="Error" w478 {
        tunnel: w477 -> [w479 w480]
        frame No Error {
          n168 = invoke class="VI" method="FP.Close"(reference=w479) -> ()  [unwired: 2 in, 3 out]
        }
        frame Error {
          n169 = invoke class="VI" method="FP.Open"(reference=w480, "Activate"=TRUE ("Activate?")) -> ()  [unwired: 3 in, 5 out]
        }
      }
    }
  }
